vi "Segment_f.vi"(11 "Input Iin Binary":bool[](array[boolean])) -> (3 "Segment f":bool)   [LabVIEW 2024]
panel:
  out "D":bool
  out "C":bool
  out "B":bool
  out "A":bool
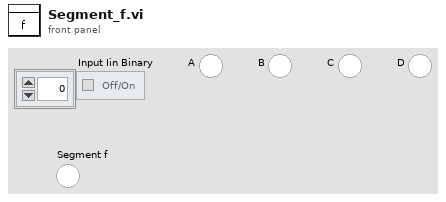
[diagram p1: front panel]
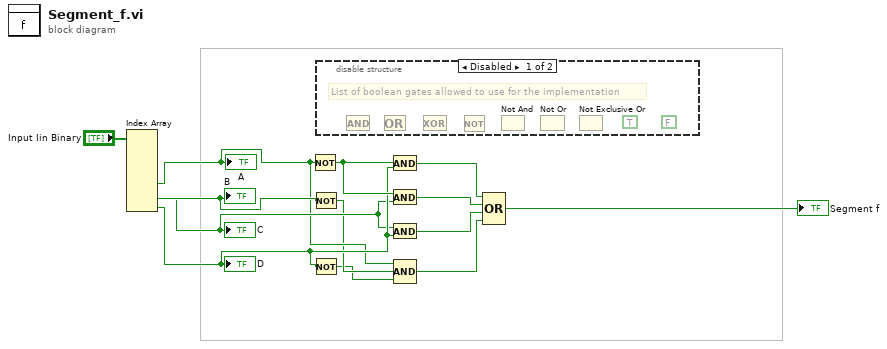
[diagram p0: block diagram]
diagram:
  n1 = Index Array(array="Input Iin Binary") -> (element #5=w8:bool, element #6=w12:bool, element #7=w9:bool, element #8=w10:bool)  [unwired: 8 in, 4 out]
  "A" <- w8
  "B" <- w12
  "C" <- w9
  "D" <- w10
  n2 = Not(x=w8) -> (.not. x?=w11:bool)
  n3 = Not(x=w12) -> (.not. x?=w7:bool)
  n4 = Not(x=w10) -> (.not. x?=w6:bool)
  n5 = disable-structure shown="Disabled" {
    frame Disabled {
      (unwired) FALSE
      (unwired) TRUE
      # "List of boolean gates allowed to use for the implementation"
      n6 = And() -> ()  [unwired: 2 in, 1 out]
      n7 = Or() -> ()  [unwired: 2 in, 1 out]
      n8 = Exclusive Or() -> ()  [unwired: 2 in, 1 out]
      n9 = Not() -> ()  [unwired: 1 in, 1 out]
      n10 = Not And() -> ()  [unwired: 2 in, 1 out]
      n11 = Not Or() -> ()  [unwired: 2 in, 1 out]
      n12 = Not Exclusive Or() -> ()  [unwired: 2 in, 1 out]
    }
    frame Enabled {
    }
  }
  n13 = And(x=w11, y=w10) -> (x .and. y?=w5:bool)
  n14 = And(x=w11, y=w9) -> (x .and. y?=w4:bool)
  n15 = And(x=w9, y=w10) -> (x .and. y?=w3:bool)
  n16 = Compound Arithmetic op=AND(w8, w7, w6) -> (w2:bool)
  n17 = Compound Arithmetic op=OR(w5, w4, w3, w2) -> (→"Segment f":bool)
